vi "8.6CompatibleGlobalVar.vi"() -> ()   [LabVIEW 2023]
panel:
  out "8.6 compatible ?":bool
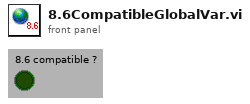
[diagram p1: front panel]
diagram:
